vi "daq_channel_read.vi"(0 "DAQmxTaskIn":refnum<k21>, 1 "chanellParaCluster":T3={"audioOffState_V"=-0.00390625, "audioFilterPeriod_uS"=500, "audioThreshold_V"=0.001953125, "vsThreshold_V"=2.0, "vsFilterPeriod_uS"=500, "lickThreshold_V"=0.0} {"vsFilterPeriod_uS" format="%#1.6f"; "audioFilterPeriod_uS" format="%#1.6f"}, 2 "error in (no error)":errorcluster) -> (3 "DAQmxTaskOut":refnum<k21>, 4 "channelOutCluster":T2, 5 "channelOutCluster_rawData":T1, 6 "error out":errorcluster)   [LabVIEW 2014]
uses:
  daq_channel_read_parameter.ctl
  <vilib>/DAQmx/read.llb/DAQmx Read (Analog 1D DBL NChan 1Samp).vi
  <vilib>/DAQmx/miscellaneous.llb/DAQmx Fill In Error Info.vi
panel:
  # "Output"
  # "Input"
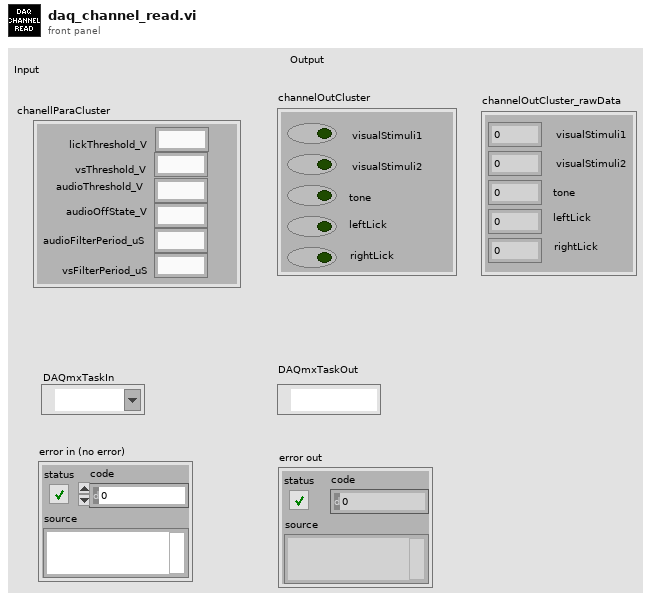
[diagram p1: front panel]
types:
  T1 = cluster{"leftLick":dbl, "rightLick":dbl, "visualStimuli2":dbl, "tone":dbl, "visualStimuli1":dbl}
  T2 = cluster{"leftLick":bool, "rightLick":bool, "visualStimuli2":bool, "tone":bool, "visualStimuli1":bool}
  T3 = typedef "daq_channel_read_parameter.ctl" = cluster{"audioOffState_V":fxp<+/-,16,5>, "audioFilterPeriod_uS":i32, "audioThreshold_V":fxp<+/-,16,5>, "vsThreshold_V":fxp<+/-,16,5>, "vsFilterPeriod_uS":i32, "lickThreshold_V":fxp<+/-,16,5>}
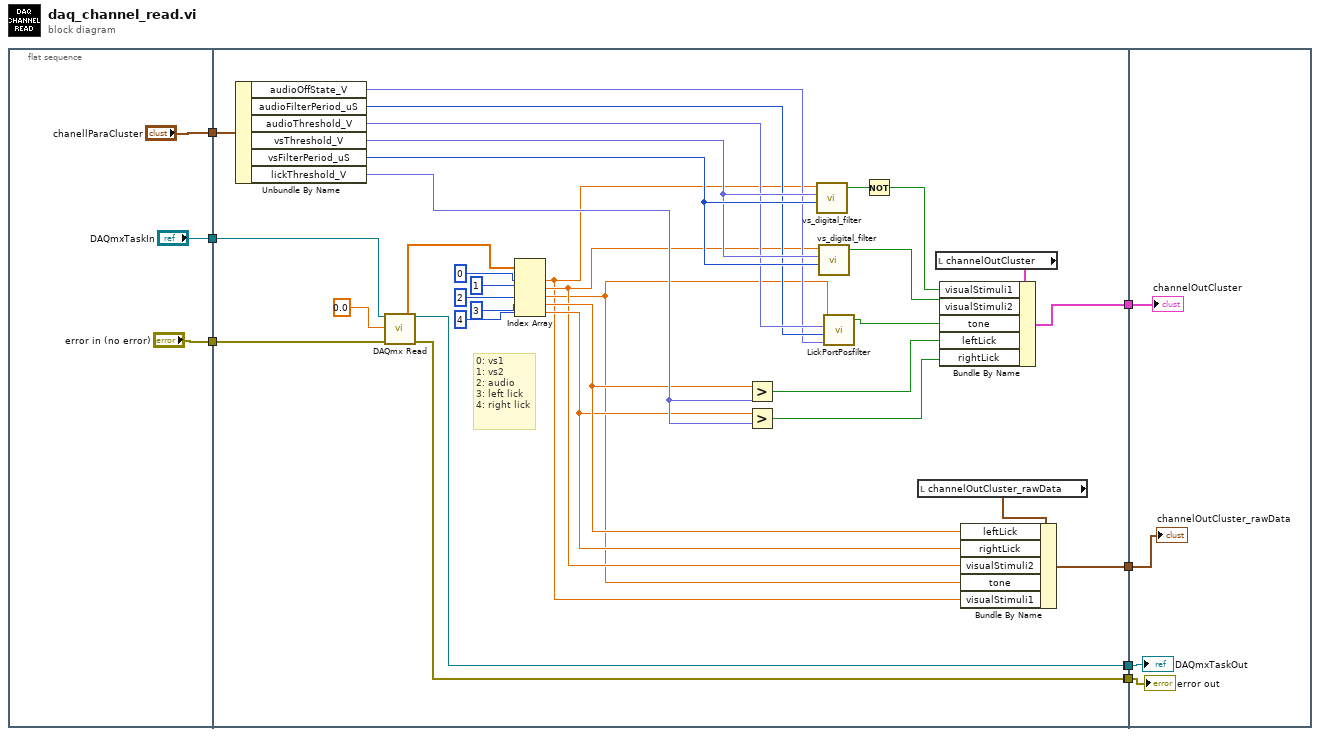
[diagram p0: block diagram]
diagram:
  n1 = flat-sequence {
    tunnel: ["DAQmxTaskIn"] -> w4
    tunnel: ["error in (no error)"] -> w3
    tunnel: ["chanellParaCluster"] -> w2
    tunnel: [w32] -> w7
    tunnel: [w31] -> w6
    tunnel: [w30] -> w5
    tunnel: w4 -> [w29]
    tunnel: w3 -> [w28]
    tunnel: w2 -> [w27]
    tunnel: [w19] -> w1
    tunnel: w7 -> [w47]
    tunnel: w6 -> [w46]
    tunnel: w5 -> [w45]
    tunnel: w1 -> [w44]
    frame #0 {
    }
    frame #1 {
      # "0: vs1\n1: vs2\n2: audio\n3: left lick\n4: right lick"
      n2 = Unbundle By Name(w27) -> ("audioOffState_V"=w21:fxp<+/-,16,5>, "audioFilterPeriod_uS"=w22:i32, "audioThreshold_V"=w23:fxp<+/-,16,5>, "vsThreshold_V"=w24:fxp<+/-,16,5>, "vsFilterPeriod_uS"=w25:i32, "lickThreshold_V"=w26:fxp<+/-,16,5>)
      n3 = call-poly <vilib>:"DAQmx Read.vi"("task/channels in"=w29, "timeout"=0.0, "error in"=w28) -> ("task out"=w31:refnum<k21>, "data"=w37:dbl[], "error out"=w30:errorcluster)  [unwired: 10 in]
      n4 = Index Array(array=w37, index #1=0, index #2=1, index #3=2, index #4=3, index #5=4) -> (element #1=w14:dbl, element #2=w16:dbl, element #3=w15:dbl, element #4=w18:dbl, element #5=w17:dbl)
      n5 = Greater?(x=w18, y=w26) -> (0:w34:bool)
      n6 = Greater?(x=w17, y=w26) -> (0:w33:bool)
      n7 = call "vs_digital_filter.vi"("filter period(uSec)"=w25, "vs threshold"=w24, "input"=w14) -> ("output"=w13:bool)  [unwired: 3 in]
      n8 = call "vs_digital_filter.vi"("filter period(uSec)"=w25, "vs threshold"=w24, "input"=w16) -> ("output"=w35:bool)  [unwired: 3 in]
      n9 = call "LickPortPosfilter.vi"("audio off state (V)"=w21, "audio filter period(uSec)"=w22, "audio threshold"=w23, "input"=w15) -> ("output"=w11:bool)  [unwired: 2 in]
      n10 = Not(x=w13) -> (.not. x?=w12:bool)
      n11 = local read "channelOutCluster_rawData"() -> (w20:T1)
      n12 = local read "channelOutCluster"() -> (w36:T2)
      n13 = Bundle By Name(cluster=w36, "visualStimuli1"=w12, "visualStimuli2"=w35, "tone"=w11, "leftLick"=w34, "rightLick"=w33) -> (w32:T2)
      n14 = Bundle By Name(cluster=w20, "leftLick"=w18, "rightLick"=w17, "visualStimuli2"=w16, "tone"=w15, "visualStimuli1"=w14) -> (w19:T1)
    }
    frame #2 {
      "DAQmxTaskOut" <- w46
      "error out" <- w45
      "channelOutCluster" <- w47
      "channelOutCluster_rawData" <- w44
    }
  }
